vi "Save synergy.vi"(3 "Synergy data":string, 5 "Step":dbl, 7 "Animal Number":dbl, 8 "Angle-angle synergygrap":i32[][](array[numeric]), 9 "Synergy Graph":i32[][](array[numeric]), 10 "Angle-angle synergy":dbl[][](array[numeric]), 11 "Synergy%":i32[][](array[numeric])) -> ()   [LabVIEW 2020]
panel:
  out "concatenated string 2":string
  out "Synergy graphs":i32[][](array[numeric])
  out "Synergy Data":dbl[][](array[numeric])
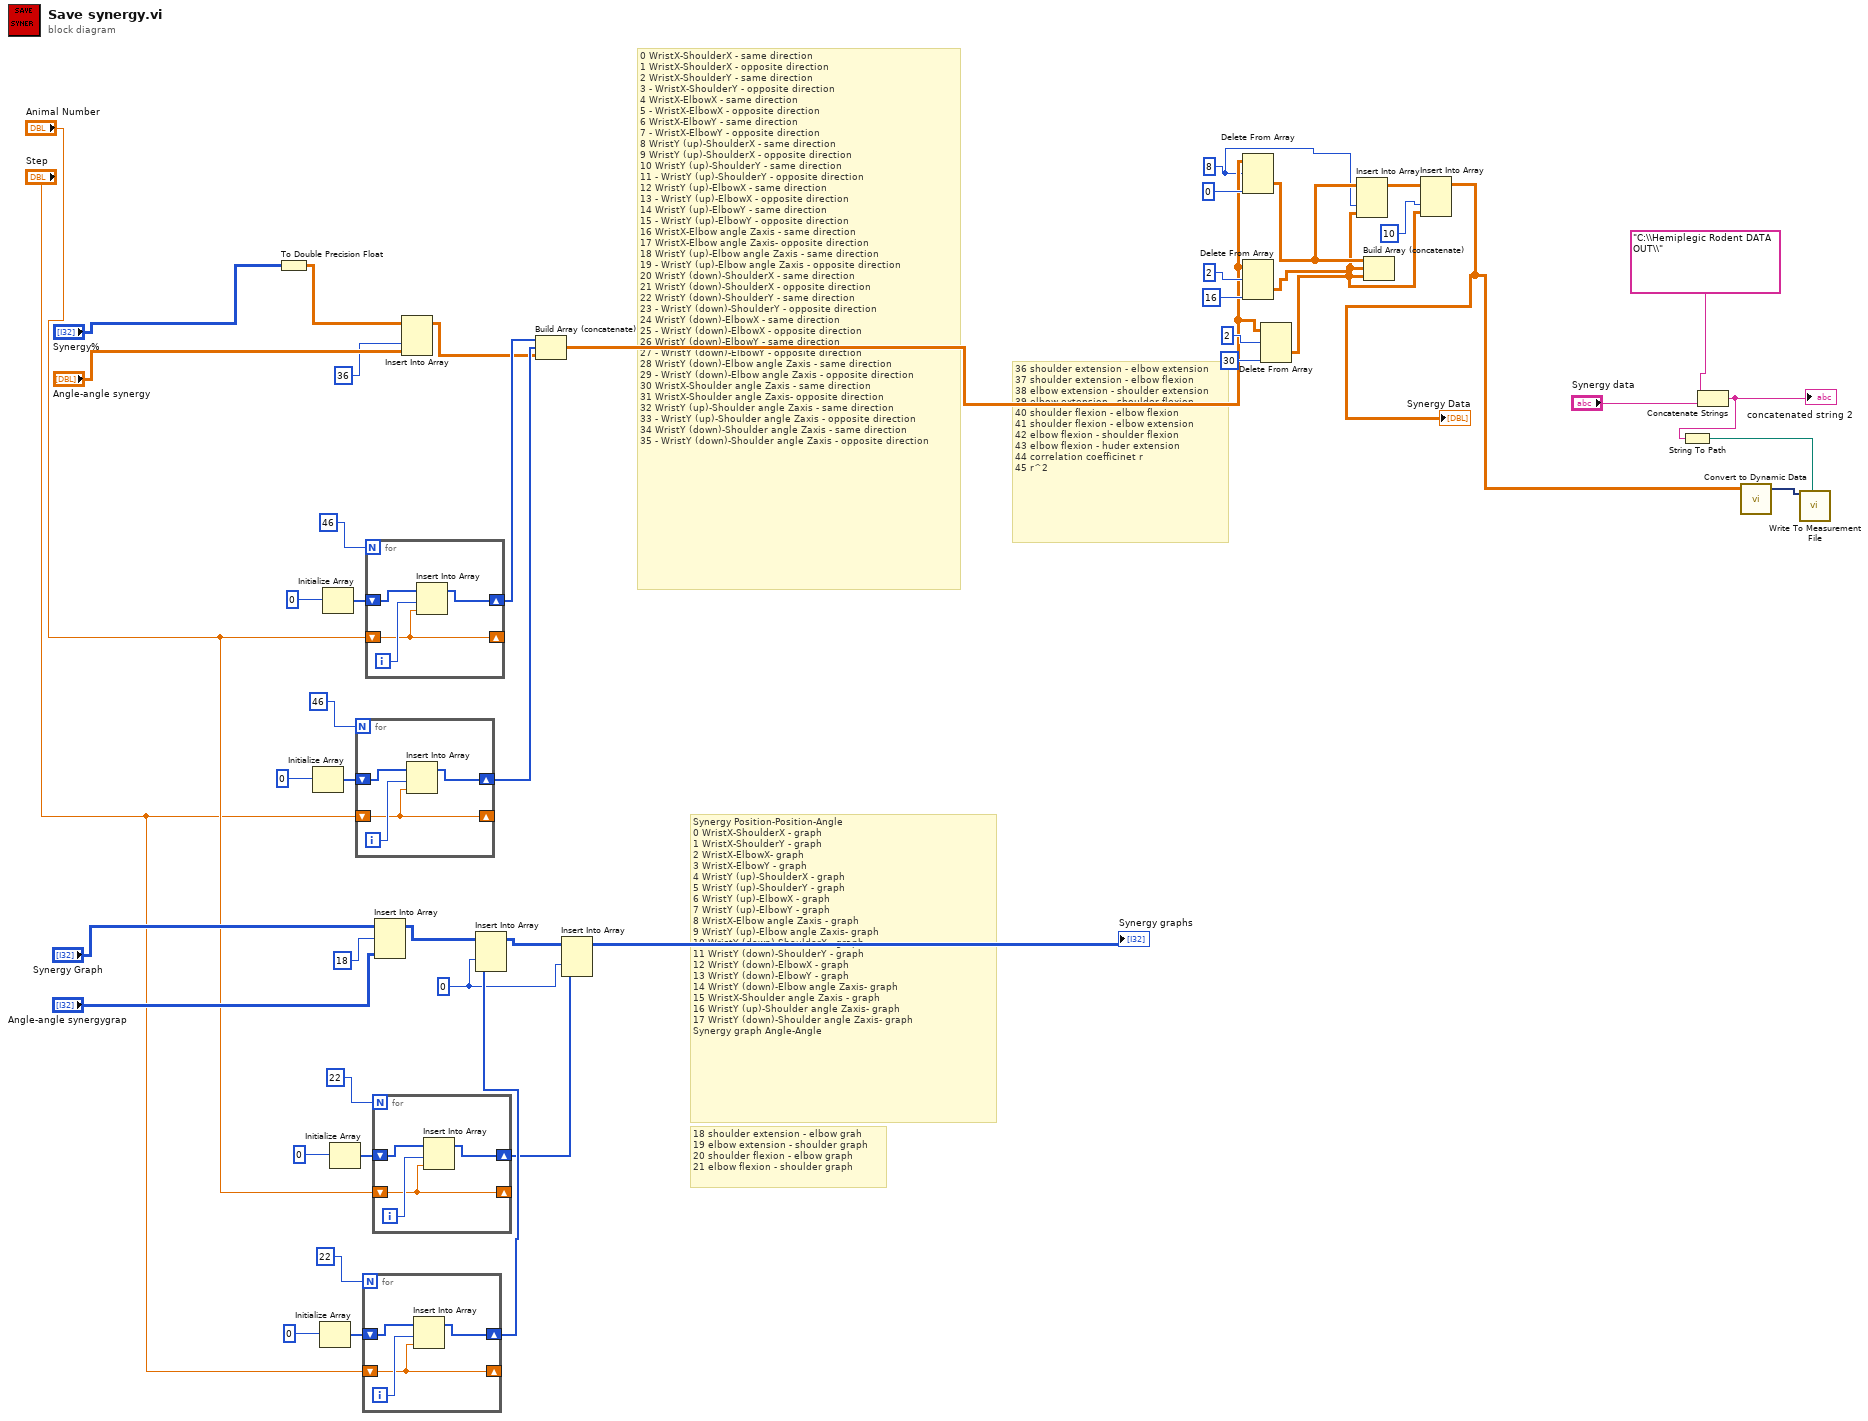
[diagram p0: block diagram]
diagram:
  w2 = 8
  w24 = 0
  # "18 shoulder extension - elbow grah\n19 elbow extension - shoulder graph\n20 shoulder flexion - elbow graph\n21 elbow flexion - shoulder graph"
  # "Synergy Position-Position-Angle\n0 WristX-ShoulderX - graph\n1 WristX-ShoulderY - graph\n2 WristX-ElbowX- graph\n3 WristX-ElbowY - graph\n4 WristY (up)-ShoulderX - graph\n5 WristY (up)-ShoulderY - graph\n6 WristY (up)-ElbowX - graph\n7 WristY (up)-ElbowY - graph\n8 WristX-Elbow angle Zaxis - graph\n9 WristY (up)-Elbow angle Zaxis- graph\n10 WristY (down)-ShoulderX - graph\n11 WristY (down)-ShoulderY - graph\n12 WristY (down)-ElbowX - graph\n13 WristY (down)-ElbowY - graph\n14 WristY (down)-Elbow angle Zaxis- graph\n15 WristX-Shoulder angle Zaxis - graph\n16 WristY (up)-Shoulder angle Zaxis- graph\n17 WristY (down)-Shoulder angle Zaxis- graph\nSynergy graph Angle-Angle"
  # "0 WristX-ShoulderX - same direction\n1 WristX-ShoulderX - opposite direction\n2 WristX-ShoulderY - same direction\n3 - WristX-ShoulderY - opposite direction\n4 WristX-ElbowX - same direction\n5 - WristX-ElbowX - opposite direction\n6 WristX-ElbowY - same direction\n7 - WristX-ElbowY - opposite direction\n8 WristY (up)-ShoulderX - same direction\n9 WristY (up)-ShoulderX - opposite direction\n10 WristY (up)-ShoulderY - same direction\n11 - WristY (up)-ShoulderY - opposite direction\n12 WristY (up)-ElbowX - same direction\n13 - WristY (up)-ElbowX - opposite direction\n14 WristY (up)-ElbowY - same direction\n15 - WristY (up)-ElbowY - opposite direction\n16 WristX-Elbow angle Zaxis - same direction\n17 WristX-Elbow angle Zaxis- opposite direction\n18 WristY (up)-Elbow angle Zaxis - same direction\n19 - WristY (up)-Elbow angle Zaxis - opposite direction\n20 WristY (down)-ShoulderX - same direction\n21 WristY (down)-ShoulderX - opposite direction\n22 WristY (down)-ShoulderY - same direction\n23 - WristY (down)-ShoulderY - opposite direction\n24 WristY (down)-ElbowX - same direction\n25 - WristY (down)-ElbowX - opposite direction\n26 WristY (down)-ElbowY - same direction\n27 - WristY (down)-ElbowY - opposite direction\n28 WristY (down)-Elbow angle Zaxis - same direction\n29 - WristY (down)-Elbow angle Zaxis - opposite direction\n30 WristX-Shoulder angle Zaxis - same direction\n31 WristX-Shoulder angle Zaxis- opposite direction\n32 WristY (up)-Shoulder angle Zaxis - same direction\n33 - WristY (up)-Shoulder angle Zaxis - opposite direction\n34 WristY (down)-Shoulder angle Zaxis - same direction\n35 - WristY (down)-Shoulder angle Zaxis - opposite direction"
  # "36 shoulder extension - elbow extension\n37 shoulder extension - elbow flexion\n38 elbow extension - shoulder extension\n39 elbow extension - shoulder flexion\n40 shoulder flexion - elbow flexion\n41 shoulder flexion - elbow extension\n42 elbow flexion - shoulder flexion\n43 elbow flexion - huder extension\n44 correlation coefficinet r\n45 r^2"
  n1 = To Double Precision Float(number="Synergy%") -> (double precision float=w36:dbl[][])
  n2 = Initialize Array(0) -> (w41:i32[])  [unwired: 1 in]
  n3 = Initialize Array(0) -> (w30:i32[])  [unwired: 1 in]
  n4 = Initialize Array(0) -> (w44:i32[])  [unwired: 1 in]
  n5 = Initialize Array(0) -> (w33:i32[])  [unwired: 1 in]
  n6 = for {
    N: 46 -> [_]
    shift-right: [w50] -> w39
    shift-left: w41 -> [w51]
    shift-right: [w49] -> _
    shift-left: "Step" -> [w49]
    i -> [w52]
    n7 = Insert Into Array(array=w51, index=w52, new element=w49) -> (w50:i32[])
  }
  n8 = for {
    N: 22 -> [_]
    shift-right: [w54] -> w25
    shift-left: w30 -> [w55]
    shift-right: [w53] -> _
    shift-left: "Step" -> [w53]
    i -> [w56]
    n9 = Insert Into Array(array=w55, index=w56, new element=w53) -> (w54:i32[])
  }
  n10 = for {
    N: 46 -> [_]
    shift-right: [w58] -> w40
    shift-left: w44 -> [w59]
    shift-right: [w57] -> _
    shift-left: "Animal Number" -> [w57]
    i -> [w60]
    n11 = Insert Into Array(array=w59, index=w60, new element=w57) -> (w58:i32[])
  }
  n12 = for {
    N: 22 -> [_]
    shift-right: [w62] -> w22
    shift-left: w33 -> [w63]
    shift-right: [w61] -> _
    shift-left: "Animal Number" -> [w61]
    i -> [w64]
    n13 = Insert Into Array(array=w63, index=w64, new element=w61) -> (w62:i32[])
  }
  n14 = Insert Into Array(array="Synergy Graph", index (row)=18, new element="Angle-angle synergygrap") -> (w26:i32[][])  [unwired: 1 in]
  n15 = Insert Into Array(array=w36, index (col)=36, new element="Angle-angle synergy") -> (w38:dbl[][])  [unwired: 1 in]
  n16 = Insert Into Array(array=w26, index (col)=w24, new element=w25) -> (w23:i32[][])  [unwired: 1 in]
  n17 = Build Array (concatenate)(w40, w39, w38) -> (w8:dbl[][])
  n18 = Insert Into Array(array=w23, index (col)=w24, new element=w22) -> (→"Synergy graphs":i32[][])  [unwired: 1 in]
  n19 = Delete From Array(array=w8, length=w2, index (col)=0) -> (deleted portion=w7:dbl[][])  [unwired: 1 in, 1 out]
  n20 = Delete From Array(array=w8, length=2, index (col)=16) -> (deleted portion=w6:dbl[][])  [unwired: 1 in, 1 out]
  n21 = Delete From Array(array=w8, length=2, index (col)=30) -> (deleted portion=w4:dbl[][])  [unwired: 1 in, 1 out]
  n22 = Insert Into Array(array=w7, index (col)=w2, new element=w6) -> (w5:dbl[][])  [unwired: 1 in]
  n23 = Build Array (concatenate)(w7, w6, w4) -> ()  [unwired: 1 out]
  n24 = Insert Into Array(array=w5, index (col)=10, new element=w4) -> (w3:dbl[][])  [unwired: 1 in]
  "Synergy Data" <- w3
  n25 = Concatenate Strings("C:\\Hemiplegic Rodent DATA OUT\\" ("name"), "Synergy data") -> (w18:string)
  "concatenated string 2" <- w18
  n26 = String To Path(string=w18) -> (path=w16:path)
  n27 = call "Convert to Dynamic Data"("2D Array"=w3) -> ("Dynamic Data Type"=w15:dynamicdata)  [unwired: 3 in]
  n28 = call "Write To Measurement File"("Signals"=w15, "Filename"=w16) -> ()  [unwired: 15 in, 3 out]
